vi "Generate pulse.vi"(10 "Pulse magnitude":dbl, 11 "Waveform parameters":T1={"Start magnitude"=0.0, "Magnitude increment"=0.0, "Number of pulses"=0, "Baseline length"=0, "Ramp length"=0, "Top  length"=0, "Threshold "=3000}) -> (2 "Data out":dbl[](array[numeric]), 3 "Waveform parameters out":T1={"Start magnitude"=0.0, "Magnitude increment"=0.0, "Number of pulses"=0, "Baseline length"=0, "Ramp length"=0, "Top  length"=0, "Threshold "=3000})   [LabVIEW 2015]
uses:
  Waveform parameters.ctl
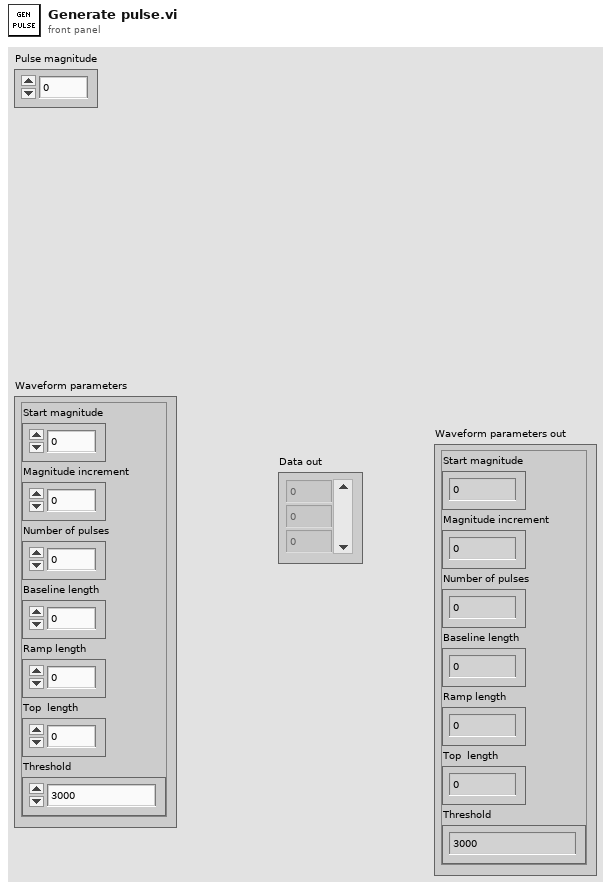
[diagram p1: front panel]
types:
  T1 = typedef "Waveform parameters.ctl" = cluster{"Start magnitude":dbl, "Magnitude increment":dbl, "Number of pulses":i32, "Baseline length":i32, "Ramp length":i32, "Top  length":i32, "Threshold ":i32}
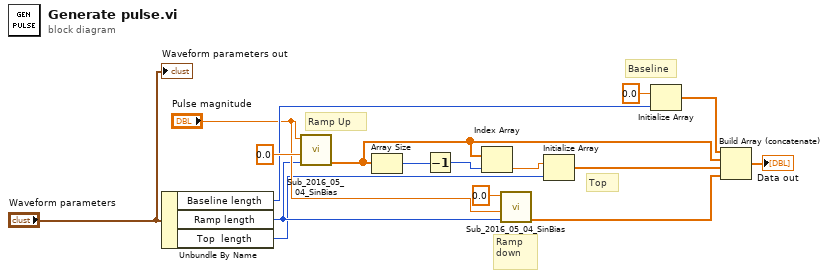
[diagram p0: block diagram]
diagram:
  # "Baseline"
  # "Ramp Up"
  # "Ramp \ndown"
  # "Top"
  n1 = Unbundle By Name("Waveform parameters") -> ("Baseline length"=w5:i32, "Ramp length"=w3:i32, "Top  length"=w2:i32)
  n2 = call "Sub_2016_05_04_SinBias.vi"("Number of steps"=w3, "Start current"=0.0, "Finish current"="Pulse magnitude") -> ("Array 2"=w7:dbl[])  [unwired: 7 in, 1 out]
  n3 = Array Size(array=w7) -> (size(s)=w6:i32)
  n4 = Decrement(x=w6) -> (x-1=w15:i32)
  n5 = Index Array(array=w7, index=w15) -> (element=w12:dbl)
  n6 = call "Sub_2016_05_04_SinBias.vi"("Number of steps"=w3, "Start current"="Pulse magnitude", "Finish current"=0.0) -> ("Array 2"=w9:dbl[])  [unwired: 7 in, 1 out]
  n7 = Initialize Array(w12, w2) -> (w10:dbl[])
  n8 = Initialize Array(0.0, w5) -> (w11:dbl[])
  n9 = Build Array (concatenate)(w11, w7, w10, w9) -> (→"Data out":dbl[])
  "Waveform parameters out" <- "Waveform parameters"
